vi "Get Items From Target.vi"(0 "Module ID":i32=-1, 2 "Local Path":string, 3 "Path on Target":string, 5 "Transfer Type":T3, 9 "Transfer Options":refnum<class "FileTransferOptions.lvclass">, 11 "error in":errorcluster, 12 "wait for reply (T)":bool=TRUE, 13 "Remove Items on Target":bool) -> (4 "Transfer Succeeded":bool, 6 "File Transfered Successfully":T2[](array[typedef]), 10 "timed out?":bool, 14 "Erroneous Transfers":T1[](array[typedef]), 15 "error out":errorcluster)   [LabVIEW 2015, in "LV-WinSCP.lvlib"]
doc: "This request allows transferring a file or an entire folder from the target to the local PC.\nFile transfer status might take longer than the module timeout. A brodacast is then also fired with the transfer status when it finishes. Therefore, asking for a reply is optional.\nA connection to the target must be done before using this request.\n_____\nCreated using DQMH Event Scripter 6.1.0.128."
uses:
  LV-WinSCP.lvlib
  Transfer Type.ctl
  Classes/FileTransferOptions/FileTransferOptions.lvclass
  Classes/FileTransfer/FileAndDestination.ctl
  Classes/FileTransfer/TransferExceptionDescription.ctl
  Get Items From Target Argument--cluster.ctl
  Get Items From Target (Reply Payload)--cluster.ctl
  Classes/FileTransfer/FileTransfer.lvclass
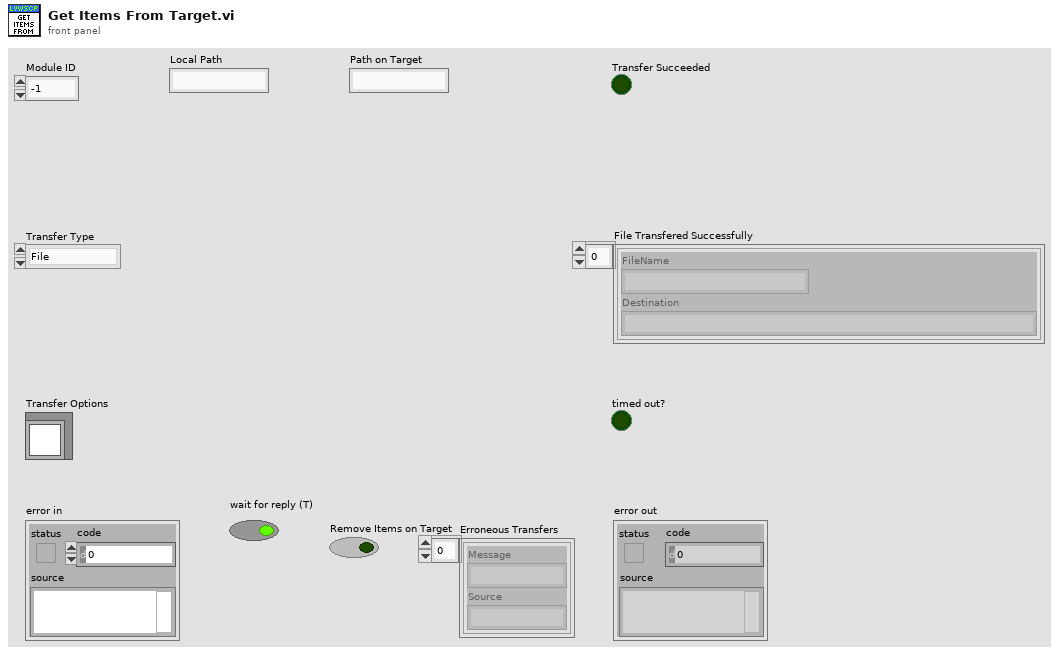
[diagram p1: front panel]
types:
  T1 = typedef "WinSCP.lvlib/FileTransfer.lvclass/TransferExceptionDescription.ctl" = cluster{"Message":string, "Source":string}
  T2 = typedef "WinSCP.lvlib/FileTransfer.lvclass/FileAndDestination.ctl" = cluster{"FileName":string, "Destination":string}
  T3 = typedef "LV-WinSCP.lvlib/Transfer Type.ctl" = enum16{"File", "Folder"}
  T4 = typedef "LV-WinSCP.lvlib/Get Items From Target Argument--cluster.ctl" = cluster{"Module ID":i32, "Transfer Type":T3, "Transfer Options":refnum<class "FileTransferOptions.lvclass">, "Wait Notifier":refnum<notifier>, "wait for reply":bool, "Path on Target":string, "Local Path":string, "Remove Items on Target":bool}
  T5 = typedef "LV-WinSCP.lvlib/Request Events--cluster.ctl" = cluster{"Stop Module":refnum<user-event>, "Show Panel":refnum<user-event>, "Hide Panel":refnum<user-event>, "Show Diagram":refnum<user-event>, "Get Module Execution Status":refnum<user-event>, "Initialize Session":refnum<user-event>, "Close Session":refnum<user-event>, "List Directory":refnum<user-event>, "Get Items From Target":refnum<user-event>}
  T6 = typedef "LV-WinSCP.lvlib/Get Items From Target (Reply Payload)--cluster.ctl" = cluster{"Transfer Succeeded":bool, "File Transfered Successfully":T2[], "Erroneous Transfers":T1[], "error":errorcluster}
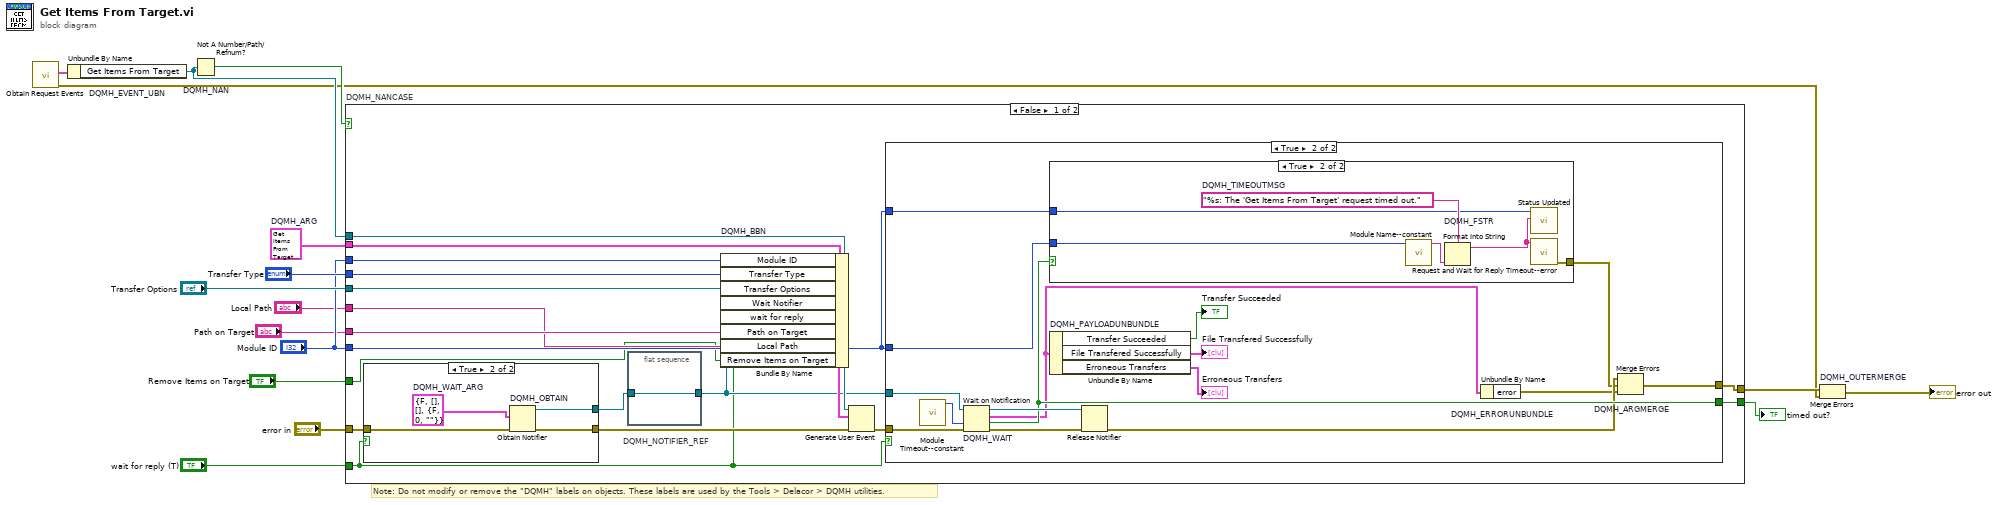
[diagram p0: block diagram]
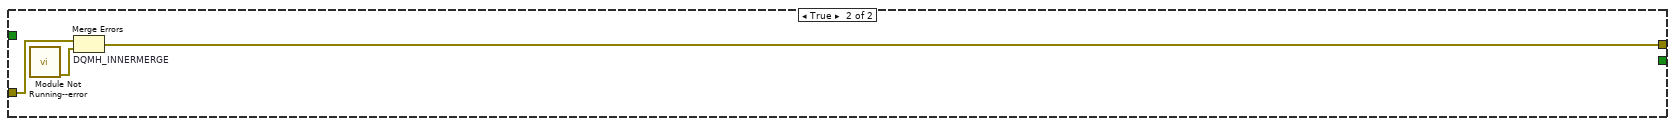
[diagram p5: hidden frame]
diagram:
  w10 = T4 {"Module ID"=-1, "Transfer Type"=enum."File", "Transfer Options"=refnum, "Wait Notifier"=refnum, "wait for reply"=FALSE, "Path on Target"="", "Local Path"="", "Remove Items on Target"=FALSE}  # DQMH_ARG
  # "Note: Do not modify or remove the \"DQMH\" labels on objects. These labels are used by the Tools > Delacor > DQMH utilities."
  n1 = call "Obtain Request Events.vi"() -> ("error out"=w5:errorcluster, "LV-WinSCP Request Events"=w4:T5)  [unwired: 10 in]
  n2 = Unbundle By Name "DQMH_EVENT_UBN"(w4) -> ("Get Items From Target"=w14:refnum<user-event>)
  n3 = Not A Number/Path/Refnum? "DQMH_NAN"(number/path/refnum=w14) -> (NaN/Path/Refnum?=w13:bool)
  n4 = case "DQMH_NANCASE" shown="False" w13 {
    tunnel: "error in" -> [w34 w66]
    tunnel: w14 -> [w32 _]
    tunnel: [w29 w65] -> w11
    tunnel: [w30 _] -> w12
    tunnel: w10 -> [w25 _]
    tunnel: "Module ID" -> [w24 _]
    tunnel: "Transfer Type" -> [w23 _]
    tunnel: "Transfer Options" -> [w22 _]
    tunnel: "Module ID" -> [w21 _]
    tunnel: "wait for reply (T)" -> [w20 _]
    tunnel: "Path on Target" -> [w19 _]
    tunnel: "Local Path" -> [w18 _]
    tunnel: "Remove Items on Target" -> [w17 _]
    frame False {
      n5 = case shown="True" w20 {
        tunnel: w34 -> [w59 w63]
        tunnel: [w59 w62] -> w31
        tunnel: [_ w60] -> w27
        frame False {
        }
        frame True {
          w61 = T6 {"Transfer Succeeded"=FALSE, "File Transfered Successfully"=[], "Erroneous Transfers"=[], "error"={"status"=FALSE, "code"=0, "source"=""}}  # DQMH_WAIT_ARG
          n6 = Obtain Notifier "DQMH_OBTAIN"(notification data type=w61, error in (no error)=w63) -> (notifier out=w60:refnum<notifier>, error out=w62:errorcluster)  [unwired: 2 in, 1 out]
        }
      }
      n7 = flat-sequence "DQMH_NOTIFIER_REF" {
        tunnel: w27 -> [w35]
        tunnel: [w35] -> w26
        frame #0 {
        }
      }
      n8 = Bundle By Name "DQMH_BBN"(cluster=w25, "Module ID"=w24, "Transfer Type"=w23, "Transfer Options"=w22, "Wait Notifier"=w26, "wait for reply"=w20, "Path on Target"=w19, "Local Path"=w18, "Remove Items on Target"=w17) -> (w28:T4)
      n9 = Generate User Event(user event=w32, event data cluster=w28, error in=w31) -> (error out=w33:errorcluster)  [unwired: 1 in, 1 out]
      n10 = case shown="True" w20 {
        tunnel: w33 -> [w36 w52]
        tunnel: w26 -> [_ w51]
        tunnel: [_ w49] -> w30
        tunnel: [w36 w48] -> w29
        tunnel: w21 -> [_ w38]
        tunnel: w21 -> [_ w37]
        frame False {
        }
        frame True {
          n11 = call "Module Timeout--constant.vi"() -> ("Module Timeout"=w42:i32)  [unwired: 11 in]
          n12 = Wait on Notification "DQMH_WAIT"(notifier=w51, timeout in ms (-1)=w42, error in (no error)=w52) -> (notifier out=w50:refnum<notifier>, notification=w43:T6, timed out?=w49:bool, error out=w47:errorcluster)  [unwired: 1 in]
          n13 = case shown="True" w49 {
            tunnel: [_ w56] -> w44
            tunnel: w38 -> [_ w54]
            tunnel: w37 -> [_ w53]
            frame False {
            }
            frame True {
              w58 = "%s: The 'Get Items From Target' request timed out."  # DQMH_TIMEOUTMSG
              n14 = call "Module Name--constant.vi"("Module ID"=w53) -> ("Module Name"=w55:string)  [unwired: 10 in]
              n15 = Format Into String "DQMH_FSTR"(format string=w58, w55) -> (resulting string=w57:string)  [unwired: 2 in, 1 out]
              n16 = call "Status Updated.vi"("Status"=w57, "Module ID"=w54) -> ()  [unwired: 9 in, 1 out]
              n17 = call "Request and Wait for Reply Timeout--error.vi"("Error Message"=w57) -> ("error out"=w56:errorcluster)  [unwired: 10 in]
            }
          }
          n18 = Unbundle By Name "DQMH_PAYLOADUNBUNDLE"(w43) -> ("Transfer Succeeded"=→"Transfer Succeeded":bool, "File Transfered Successfully"=→"File Transfered Successfully":T2[], "Erroneous Transfers"=→"Erroneous Transfers":T1[])
          n19 = Release Notifier(notifier=w50, error in (no error)=w47) -> (error out=w46:errorcluster)  [unwired: 1 in, 2 out]
          n20 = Unbundle By Name "DQMH_ERRORUNBUNDLE"(w43) -> ("error"=w45:errorcluster)
          n21 = Merge Errors "DQMH_ARGMERGE"(w46, w44, w45) -> (w48:errorcluster)
        }
      }
    }
    frame True {
      n22 = call "Module Not Running--error.vi"() -> ("error out"=w64:errorcluster)  [unwired: 11 in]
      n23 = Merge Errors "DQMH_INNERMERGE"(w66, w64) -> (w65:errorcluster)
    }
  }
  "timed out?" <- w12
  n24 = Merge Errors "DQMH_OUTERMERGE"(w11, w5) -> (→"error out":errorcluster)
